vi "specs_test.vi"() -> ()   [LabVIEW 2020]
uses:
  subvi/ProdigyRemoteControlLib/DEFINITIONS/DEF_SpectrumParaInfo.ctl
  subvi/ProdigyRemoteControlLib/ProdigyRemoteControl.lvlib
panel:
  in  "Combo Box":string(combo)
  out "Scan Range":T1
  out "Lens Modes":T1
  out "Analyzer Parameter Values":string[](array[string])
  out "Analyzer Parameter Names":string[](array[string])
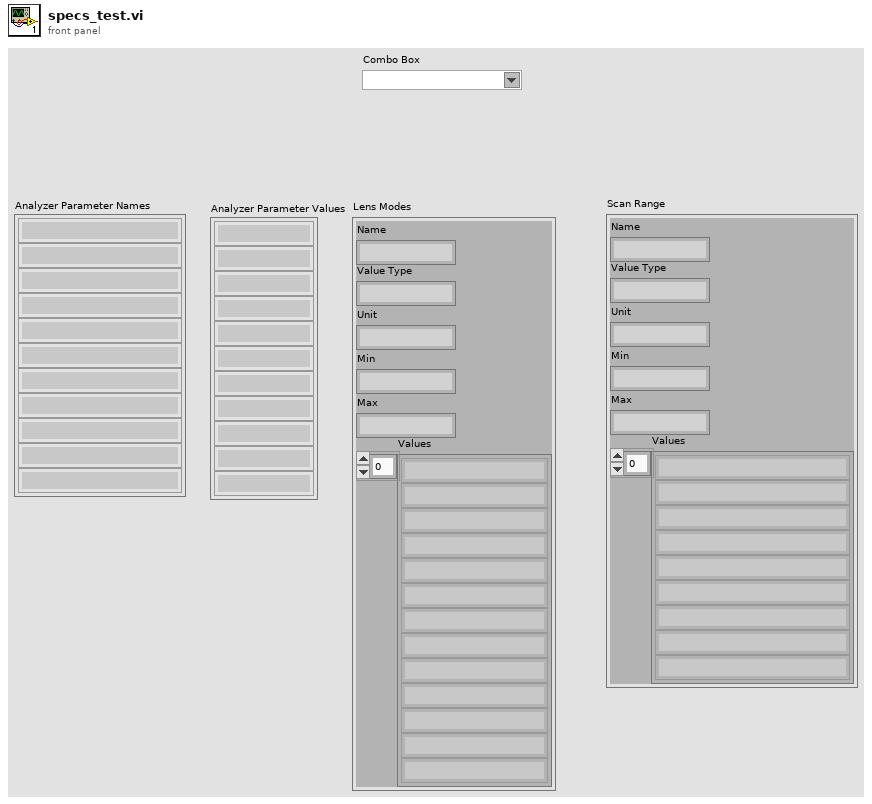
[diagram p1: front panel]
types:
  T1 = typedef "ProdigyRemoteControl.lvlib/DEF_SpectrumParaInfo.ctl" = cluster{"Name":string, "Value Type":string, "Unit":string, "Min":string, "Max":string, "Values":string[]}
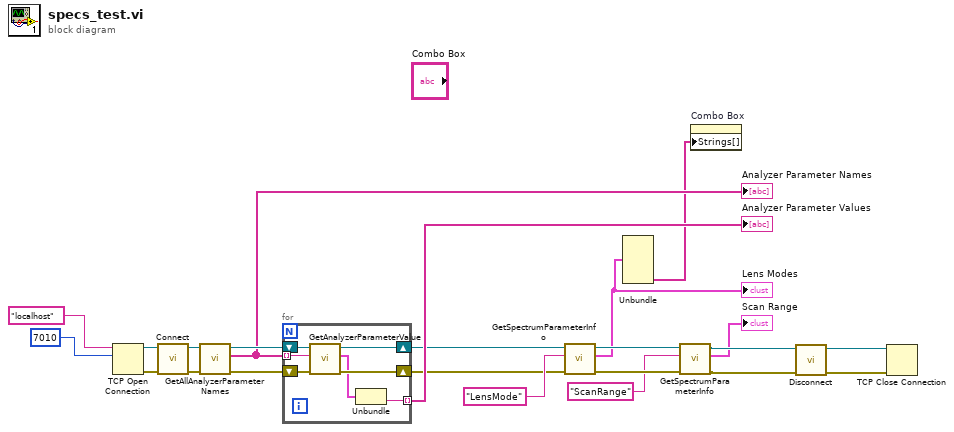
[diagram p0: block diagram]
diagram:
  n1 = TCP Open Connection(address="localhost", remote port or service name=u16 7010) -> (connection ID=w21:refnum<k5>, error out=w20:errorcluster)  [unwired: 3 in]
  n2 = call "Connect.vi"("error in"=w20, "connection ID in"=w21) -> ("error out"=w18:errorcluster, "connection ID out"=w19:refnum<k5>)  [unwired: 4 in, 4 out]
  n3 = call "GetAllAnalyzerParameterNames.vi"("error in"=w18, "connection ID in"=w19) -> ("error out"=w14:errorcluster, "Analyzer Parameter Names"=w13:string[], "connection ID out"=w15:refnum<k5>)  [unwired: 4 in, 3 out]
  "Analyzer Parameter Names" <- w13
  n4 = for {
    shift-right: [w29] -> w4
    shift-left: w15 -> [w30]
    shift-right: [w28] -> w3
    shift-left: w14 -> [w27]
    tunnel: w13 -> [w26] mode=indexing
    tunnel: [w24] -> w12 mode=indexing
    n5 = call "GetAnalyzerParameterValue.vi"("error in"=w27, "Parameter Name"=w26, "connection ID in"=w30) -> ("error out"=w28:errorcluster, "Parameter"=w25:cluster{"Name":string, "Value":string}, "connection ID out"=w29:refnum<k5>)  [unwired: 3 in, 3 out]
    n6 = Unbundle(w25) -> ("Value"=w24:string)  [unwired: 1 out]
  }
  "Analyzer Parameter Values" <- w12
  n7 = call "GetSpectrumParameterInfo.vi"("error in"=w3, "Parameter Name"="LensMode", "connection ID in"=w4) -> ("error out"=w9:errorcluster, "Spectrum Parameter Info"=w2:T1, "connection ID out"=w10:refnum<k5>)  [unwired: 3 in, 3 out]
  "Lens Modes" <- w2
  n8 = Unbundle(w2) -> ("Values"=w1:string[])  [unwired: 5 out]
  n9 = call "GetSpectrumParameterInfo.vi"("error in"=w9, "Parameter Name"="ScanRange", "connection ID in"=w10) -> ("error out"=w6:errorcluster, "Spectrum Parameter Info"=→"Scan Range":T1, "connection ID out"=w7:refnum<k5>)  [unwired: 3 in, 3 out]
  n10 = property on="Combo Box" class="CmbBox"("Strings[]"=w1) -> ()  [unwired: 2 in, 2 out]
  n11 = call "Disconnect.vi"("error in"=w6, "connection ID in"=w7) -> ("error out"=w16:errorcluster, "connection ID out"=w17:refnum<k5>)  [unwired: 5 in, 3 out]
  n12 = TCP Close Connection(connection ID=w17, error in (no error)=w16) -> ()  [unwired: 1 in, 2 out]
